vi "Pad Size.vi"(5 "Force Zero (F)":bool, 7 "Padding (0)":i32, 11 "Value":i32) -> (2 "Padded or Zero":i32, 3 "Value or Zero":i32)   [LabVIEW 2022 SP3, in "FlexBlocks Support.lvlib"]
uses:
  FlexBlocks Support.lvlib
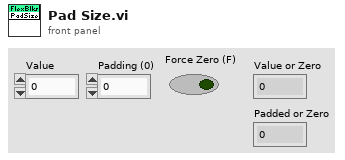
[diagram p1: front panel]
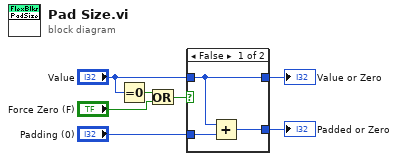
[diagram p0: block diagram]
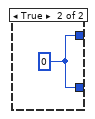
[diagram p2: hidden frame]
diagram:
  n1 = Equal To 0?(x="Value") -> (x = 0?=w7:bool)
  n2 = Or(x=w7, y="Force Zero (F)") -> (x .or. y?=w6:bool)
  n3 = case shown="False" w6 {
    tunnel: "Value" -> [w9 _]
    tunnel: "Padding (0)" -> [w10 _]
    tunnel: [w9 w11] -> w2
    tunnel: [w8 w11] -> w1
    frame False {
      n4 = Add(x=w9, y=w10) -> (x+y=w8:i32)
    }
    frame True {
      w11 = 0 ("Value")
    }
  }
  "Value or Zero" <- w2
  "Padded or Zero" <- w1
